vi "instrumentProperties_channel_attenuatorAvailable.vi"(8 "error in (no error)":errorcluster, 11 "OSAchannel in":refnum<class "OSAchannel.lvclass">) -> (0 "error out":errorcluster, 2 "attenuationFilterAvailable":bool, 3 "OSAchannel out":refnum<class "OSAchannel.lvclass">)   [LabVIEW 2010, in "OSAchannel.lvclass"]
uses:
  OSAchannel.lvclass
  OSAchannel.lvclass/OSAchannel.ctl
  FTSLib.dll
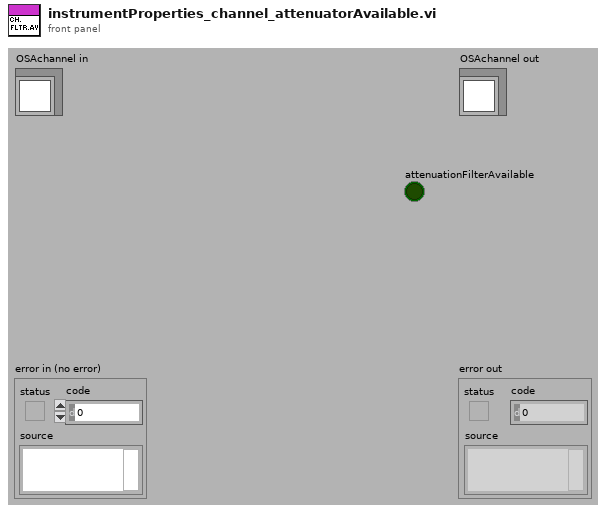
[diagram p1: front panel]
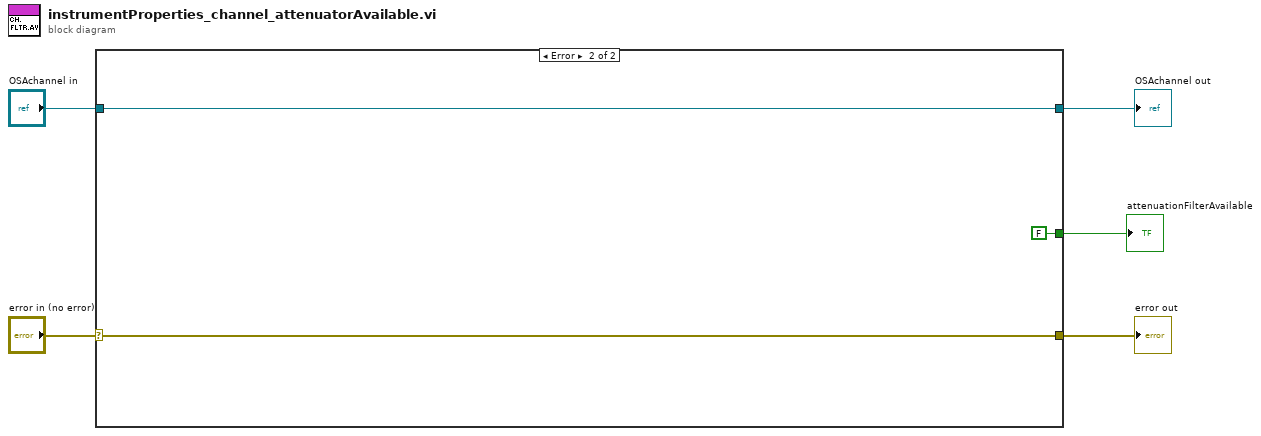
[diagram p0: block diagram]
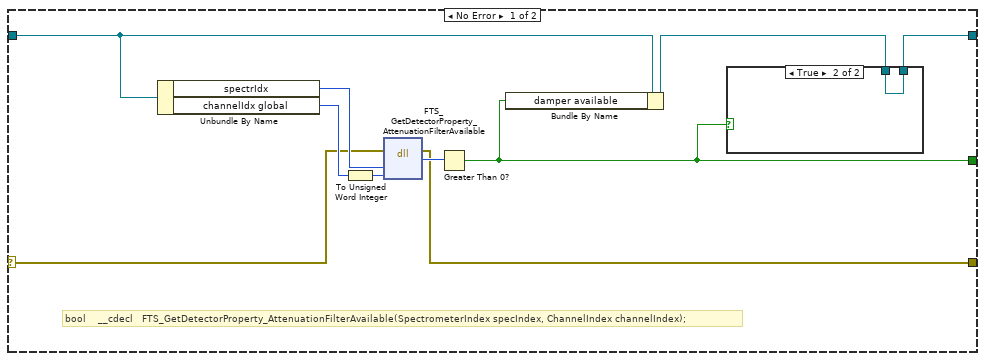
[diagram p2: hidden frame]
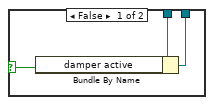
[diagram p3: hidden frame]
diagram:
  n1 = case shown="Error" "error in (no error)" {
    selector: "error in (no error)" -> [w12 w22]
    tunnel: [w9 w22] -> w4
    tunnel: [w6 w21] -> w2
    tunnel: "OSAchannel in" -> [w11 w21]
    tunnel: [w8 FALSE] -> w1
    frame No Error {
      # "bool \t\t\t__cdecl   FTS_GetDetectorProperty_AttenuationFilterAvailable(SpectrometerIndex specIndex, ChannelIndex channelIndex);"
      n2 = Unbundle By Name(w11) -> ("spectrIdx"=w15:u16, "channelIdx global"=w14:u16)
      n3 = To Unsigned Word Integer(number=w14) -> (unsigned 16bit integer=w13:u16)
      n4 = dll-call lib="FTSLib.dll" fn="FTS_GetDetectorProperty_AttenuationFilterAvailable"(error in=w12, "spectrIdx"=w15, "channeldx"=w13) -> (error out=w9:errorcluster, "filterAvailable"=w10:i32)  [unwired: 4 in, 1 out]
      n5 = Greater Than 0?(x=w10) -> (x > 0?=w8:bool)
      n6 = Bundle By Name(cluster=w11, "damper available"=w8) -> (w7:refnum<class "OSAchannel.lvclass">)
      n7 = case shown="True" w8 {
        selector: w8 -> [w17 _]
        tunnel: w7 -> [w18 w19]
        tunnel: [w16 w19] -> w6
        frame False {
          n8 = Bundle By Name(cluster=w18, "damper active"=w17) -> (w16:refnum<class "OSAchannel.lvclass">)
        }
        frame True {
        }
      }
    }
    frame Error {
    }
  }
  "error out" <- w4
  "OSAchannel out" <- w2
  "attenuationFilterAvailable" <- w1
